vi "Test Table class.vi"() -> ()   [LabVIEW 2011]
uses:
  stats.lvclass
panel:
  in  "Tree":string(tree)
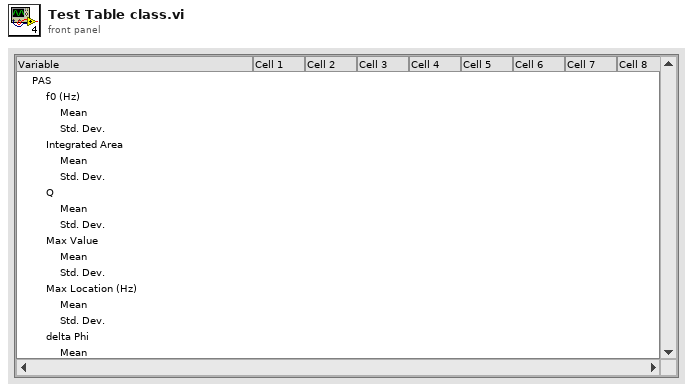
[diagram p1: front panel]
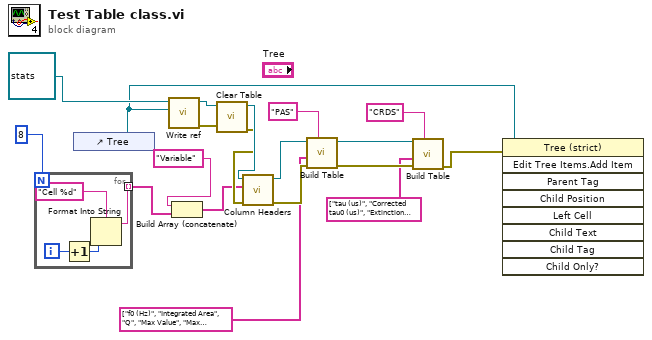
[diagram p0: block diagram]
diagram:
  n1 = for {
    N: 8 -> [_]
    tunnel: [w20] -> w10 mode=indexing
    i -> [w22]
    n2 = Increment(x=w22) -> (x+1=w21:i32)
    n3 = Format Into String(format string="Cell %d", w21) -> (resulting string=w20:string)  [unwired: 2 in, 1 out]
  }
  n4 = control-ref of="Tree"() -> (w2:refnum<vi>)
  n5 = call "Write ref.vi"("ref"=w2, "stats in"=refnum<class "stats.lvclass"> refnum ("stats.lvclass")) -> ("error out"=w16:errorcluster, "stats out"=w17:refnum<class "stats.lvclass">)  [unwired: 8 in]
  n6 = Build Array (concatenate)("Variable", w10) -> (w8:string[])
  n7 = call "Clear Table.vi"("error in (no error)"=w16, "stats in"=w17) -> ("error out"=w13:errorcluster, "stats out"=w15:refnum<class "stats.lvclass">)  [unwired: 8 in]
  n8 = call "Column Headers.vi"("error in"=w13, "column_header"=w8, "stats in"=w15) -> ("error out"=w12:errorcluster, "stats out"=w14:refnum<class "stats.lvclass">)  [unwired: 7 in]
  n9 = call "Build Table.vi"("Instrument"="PAS", "error in"=w12, "variables"=string[] ["f0 (Hz)", "Integrated Area", "Q", "Max Value", "Max Location (Hz)", "delta Phi", "tau", "Noise Limit", "Absorbtion (Mm^-1)"] ("Y Axis Labels"), "stats in"=w14) -> ("error out"=w6:errorcluster, "stats out"=w7:refnum<class "stats.lvclass">)  [unwired: 6 in]
  n10 = call "Build Table.vi"("Instrument"="CRDS", "error in"=w6, "variables"=string[] ["tau (us)", "Corrected tau0 (us)", "Extinction (Mm-1)", "Corrected Extinction (Mm-1)", "Std. Dev. in tau (us)", "Error in tau", "Corrected tau (us)", "tau0 (us)", "Max Amplitude"], "stats in"=w7) -> ("error out"=w1:errorcluster)  [unwired: 6 in, 1 out]
  n11 = invoke class="Tree (strict)" method="Edit Tree Items.Add Item"(reference=w2, error in=w1) -> ()  [unwired: 7 in, 9 out]
